vi "Local Remote.vi"(8 "error in":errorcluster, 10 "Remote (T: Remote)":bool=TRUE, 11 "VISA resource name":refnum<visa-resource-name>) -> (0 "error out":errorcluster, 3 "VISA resource out":refnum<visa-resource-name>)   [LabVIEW 2019, in "Acopian.lvlib" / "Acopian.lvclass"]
uses:
  Library/Acopian.lvclass
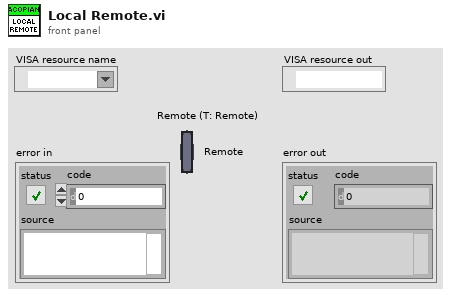
[diagram p1: front panel]
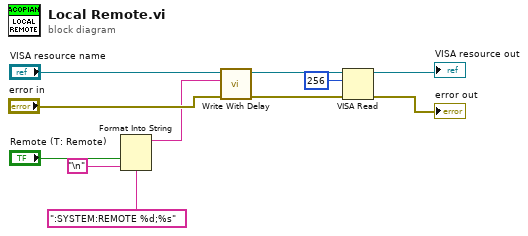
[diagram p0: block diagram]
diagram:
  n1 = Format Into String(format string=":SYSTEM:REMOTE %d;%s" ("Enable/Disable Output"), "Remote (T: Remote)", "\n") -> (resulting string=w1:string)  [unwired: 2 in, 1 out]
  n2 = call "Write With Delay.vi"("error in"="error in", "write buffer"=w1, "VISA resource name"="VISA resource name") -> ("error out"=w5:errorcluster, "VISA resource name out"=w4:refnum<visa-resource-name>)  [unwired: 7 in]
  n3 = VISA Read(VISA resource name=w4, byte count=u32 256, error in (no error)=w5) -> (VISA resource name out=→"VISA resource out":refnum<visa-resource-name>, error out=→"error out":errorcluster)  [unwired: 2 out]
